vi "Sweep - Create Tasks.vi"(8 "error in (no error)":errorcluster, 11 "measurement configuration":T3={"digital channel list"="", "frame clock rate"=0.0, "number of channels"=0, "channel length"=0, "bit depth"=0, "data justification"=enum."Left Justified", "endianness"=enum."MSB First", "bit clock edge sync"=enum."Rising", "frame sync edge for channel 0"=enum."Rising", "channel 0 offset"=0, "master clock channel list"="", "master clock rate"=0.0, "enable dither"=FALSE, "logic level"=enum."3.3 V", "signal frequency"=1000.0, "output level"=0.0, "output level units"=enum."% FS", "output range (pk-pk)"=0.0, "load impedance"=0.0, "signal phase"=0.0, "acq sampling rate"=0.0, "min measurement cycles"=0, "min measurement time (s)"=0.0, "min settling cycles"=0, "min settling time (s)"=0.0, "acq channel"="", "band start"=0.0, "band stop"=0.0, "weighting filter"=enum."Linear", "highpass filter"=enum."DC", "lowpass filter"=enum."No filter", "SNR units"=enum."dB", "THD+N units"=enum."dB", "THD units"=enum."dB", "gain units"=enum."dB"} {"signal phase" format="%0.2f"; "master clock rate" format="%#_6pHz"; "frame clock rate" format="%#_6pHz"}) -> (0 "error out":errorcluster, 2 "DAQmx task":refnum<k21>, 3 "PCM tasks":T1)   [LabVIEW 2023]
uses:
  controls/single tone measurement settings (HW).ctl
  controls/digital audio protocol/data justification.ctl
  controls/digital audio protocol/endianness.ctl
  controls/digital audio protocol/digital edge.ctl
  controls/digital audio protocol/logic level.ctl
  controls/digital output level units.ctl
  controls/weighting filter.ctl
  controls/highpass filter.ctl
  controls/lowpass filter.ctl
  controls/units - snr.ctl
  controls/units - ratio.ctl
  controls/digital audio protocol/PCM tasks.ctl
  <vilib>/PDM Acquisition Toolkit/host/Classes/Tasks/PCM Output/Controls/PCM Output Task DVR.ctl
  <vilib>/PDM Acquisition Toolkit/host/Classes/Tasks/PCM Output/PCM Output Task.lvclass
  <vilib>/PDM Acquisition Toolkit/shared/controls/clock mode.ctl
  <vilib>/PDM Acquisition Toolkit/shared/controls/PCM Frame Sync Control.ctl
  <vilib>/PDM Acquisition Toolkit/shared/controls/Digital Edge.ctl
  <vilib>/PDM Acquisition Toolkit/shared/controls/PCM Data Format Configuration.ctl
  <vilib>/PDM Acquisition Toolkit/shared/controls/PCM Bit Endianness.ctl
  <vilib>/PDM Acquisition Toolkit/shared/controls/PCM Data Justification.ctl
  <vilib>/DAQmx/create/channels.llb/DAQmx Create Channel (AI-Voltage-Basic).vi
  <vilib>/DAQmx/configure/timing.llb/DAQmx Timing (Sample Clock).vi
  <vilib>/PDM Acquisition Toolkit/host/API/Public/Function Generator/Configure Custom Signal (N Ch) - PCM Output Task.vi
  <vilib>/PDM Acquisition Toolkit/shared/PDM Shared.lvlib
  <vilib>/PDM Acquisition Toolkit/host/API/PDM Acquisition Toolkit.lvlib
  controls/audio controls.lvlib
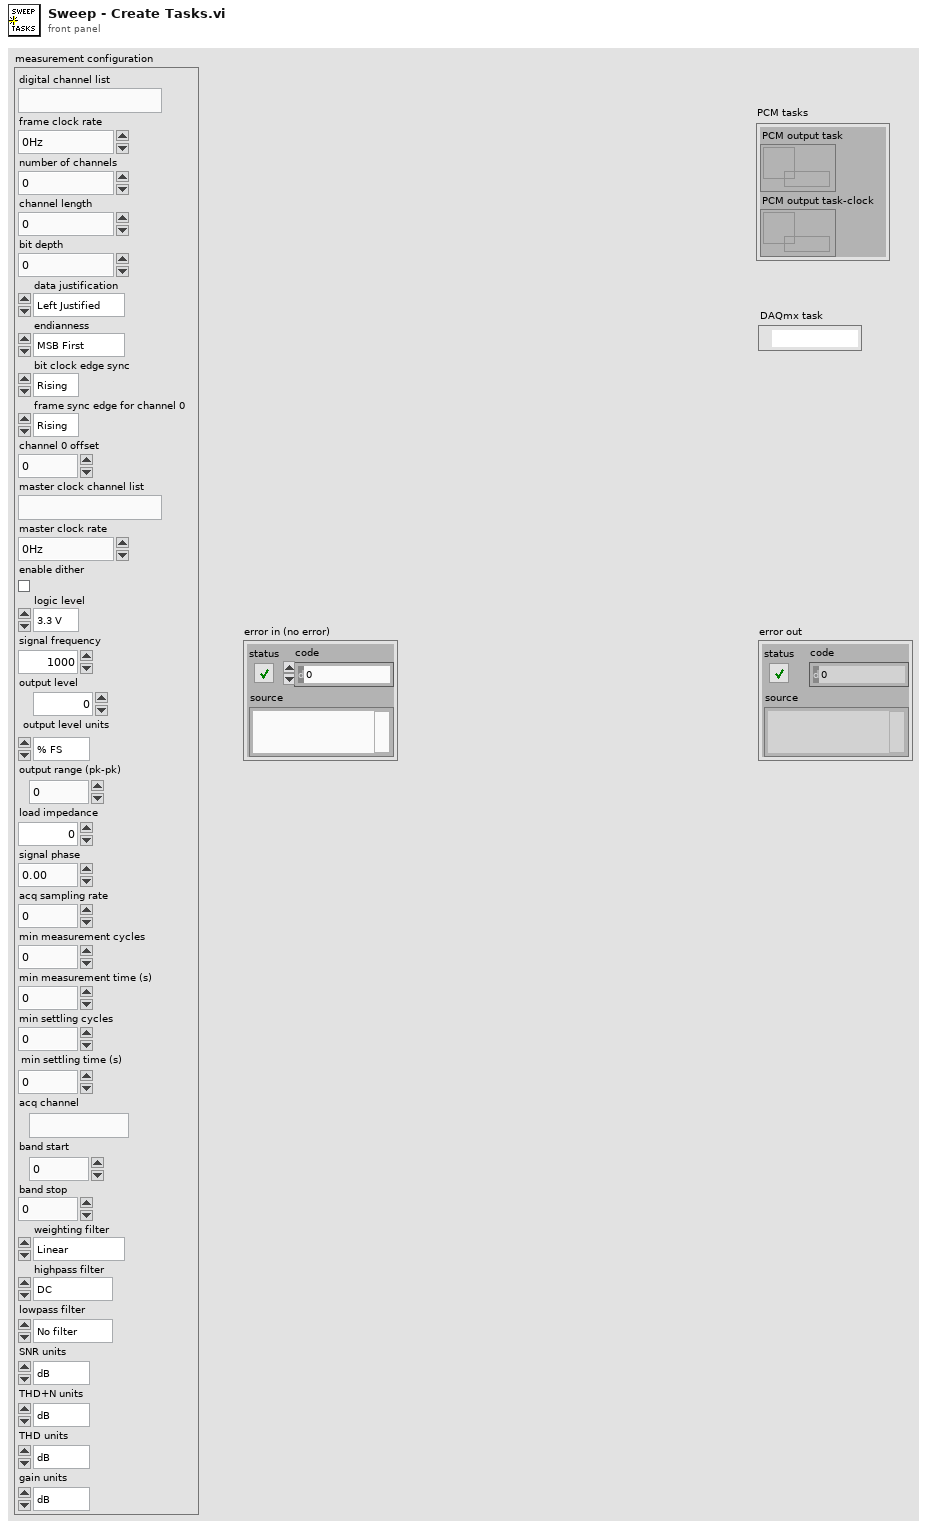
[diagram p1: front panel]
types:
  T1 = typedef "PCM tasks.ctl" = cluster{"PCM output task":T2, "PCM output task-clock":T2}
  T2 = typedef "PDM Acquisition Class Library.lvlib/PCM Output Task.lvclass/PCM Output Task DVR.ctl" = refnum<data-value>
  T3 = typedef "single tone measurement settings (HW).ctl" = cluster{"digital channel list":string, "frame clock rate":dbl, "number of channels":u32, "channel length":u32, "bit depth":u32, "data justification":T4, "endianness":T5, "bit clock edge sync":T6, "frame sync edge for channel 0":T6, "channel 0 offset":u32, "master clock channel list":string, "master clock rate":dbl, "enable dither":bool, "logic level":T7, "signal frequency":dbl, "output level":dbl, "output level units":T8, "output range (pk-pk)":dbl, "load impedance":dbl, "signal phase":dbl, "acq sampling rate":dbl, "min measurement cycles":u32, "min measurement time (s)":dbl, "min settling cycles":u32, "min settling time (s)":dbl, "acq channel":string, "band start":dbl, "band stop":dbl, "weighting filter":T9, "highpass filter":T10, "lowpass filter":T11, "SNR units":T12, "THD+N units":T13, "THD units":T13, "gain units":T13}
  T4 = typedef "data justification.ctl" = enum32{"Left Justified", "Right Justified"}
  T5 = typedef "endianness.ctl" = enum32{"MSB First", "LSB First"}
  T6 = typedef "digital edge.ctl" = enum32{"Rising", "Falling"}
  T7 = typedef "logic level.ctl" = enum32{"3.3 V", "1.8 V", "1.2 V"}
  T8 = typedef "audio controls.lvlib/digital output level units.ctl" = enum32{"% FS", "dBFS", "V"}
  T9 = typedef "weighting filter.ctl" = enum32{"Linear", "A-weighting", "B-weighting", "C-weighting"}
  T10 = typedef "highpass filter.ctl" = enum32{"DC", "AC"}
  T11 = typedef "lowpass filter.ctl" = enum32{"No filter", "AES17 20kHz", "AES17 40kHz"}
  T12 = typedef "audio controls.lvlib/units - snr.ctl" = enum32{"dB", "x/y"}
  T13 = typedef "audio controls.lvlib/units - ratio.ctl" = enum32{"dB", "%", "x/y"}
  T14 = typedef "PDM Shared.lvlib/PCM Data Format Configuration.ctl" = cluster{"Frame Sync Edge for Channel 0":T15, "Channel Count Per Frame":u8, "Channel Length":u16, "Bit Depth":u8, "Channel 0 Offset":u16, "Endianness":T16, "Data Justification":T17}
  T15 = typedef "PDM Shared.lvlib/Digital Edge.ctl" = enum8{"Rising", "Falling"}
  T16 = typedef "PDM Shared.lvlib/PCM Bit Endianness.ctl" = enum16{"MSB First", "LSB First"}
  T17 = typedef "PDM Shared.lvlib/PCM Data Justification.ctl" = enum16{"Left Justified", "Right Justified"}
  T18 = typedef "PDM Shared.lvlib/PCM Frame Sync Control.ctl" = cluster{"Frame Length":u16, "Frame Sync Pulse Width":u16, "Bit Clock Edge  Sync":T15}
  T19 = typedef "PDM Shared.lvlib/clock mode.ctl" = enum16{"divided clock", "DDS"}
  T20 = typedef "PDM Acquisition Class Library.lvlib/I2S Output Task.lvclass/SignalProperties.ctl" = cluster{"cyclic signal":dbl[], "channel parameters":T21[]}
  T21 = typedef "PDM Acquisition Class Library.lvlib/I2S Output Channel.lvclass/GenerationChannelProperties.ctl" = cluster{"cyclic period":dbl, "cyclic phase offset":dbl, "gain":dbl}
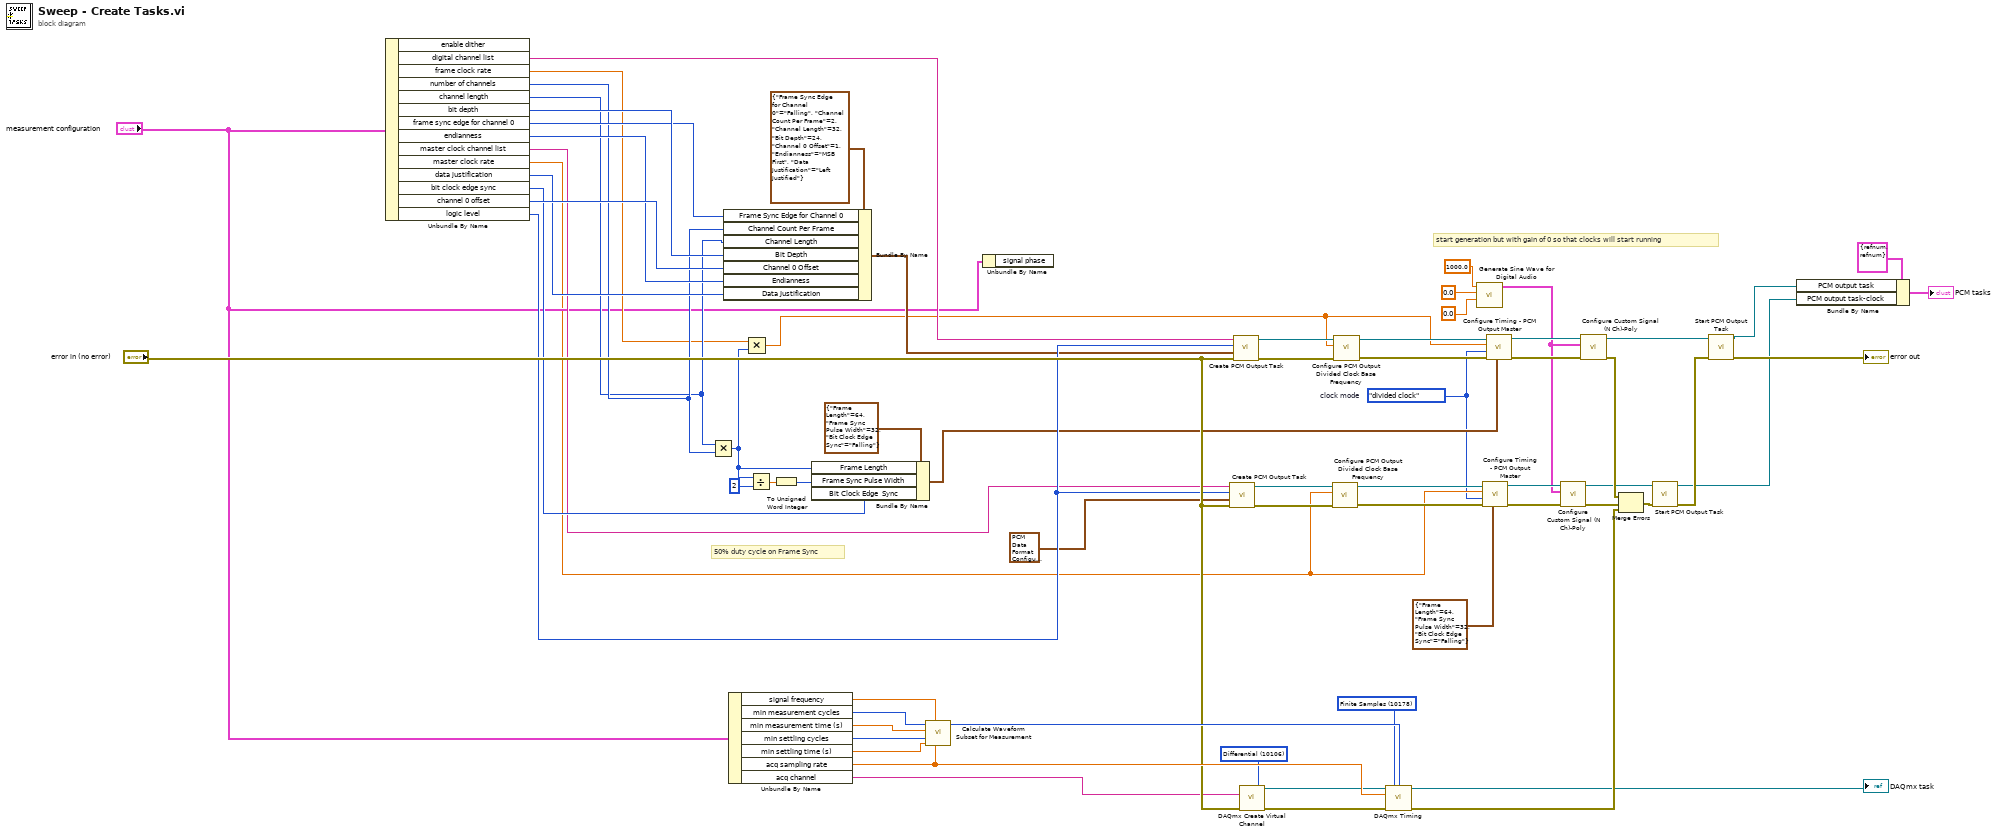
[diagram p0: block diagram]
diagram:
  w51 = 10106 items=["Default"=-1, "RSE"=10083, "NRSE"=10078, "Differential"=10106, "Pseudodifferential"=12529] ("input terminal configuration")
  w45 = 10178 items=["Finite Samples"=10178, "Continuous Samples"=10123, "Hardware Timed Single Point"=12522] ("sample mode")
  w1 = clock_mode."divided clock"  # clock mode
  # "start generation but with gain of 0 so that clocks will start running"
  # "50% duty cycle on Frame Sync"
  n1 = Unbundle By Name("measurement configuration") -> ("digital channel list"=w58:string, "frame clock rate"=w46:dbl, "number of channels"=w48:u32, "channel length"=w47:u32, "bit depth"=w68:u32, "frame sync edge for channel 0"=w53:T6, "endianness"=w54:T5, "master clock channel list"=w49:string, "master clock rate"=w2:dbl, "data justification"=w52:T4, "bit clock edge sync"=w55:T6, "channel 0 offset"=w56:u32, "logic level"=w57:T7)  [unwired: 1 out]
  n2 = Multiply(x=w47, y=w48) -> (x*y=w33:u32)
  n3 = Bundle By Name(cluster=T14 {"Frame Sync Edge for Channel 0"=enum."Falling", "Channel Count Per Frame"=2, "Channel Length"=32, "Bit Depth"=24, "Channel 0 Offset"=1, "Endianness"=enum."MSB First", "Data Justification"=enum."Left Justified"} ("PCM Data Configuration"), "Frame Sync Edge for Channel 0"=w53, "Channel Count Per Frame"=w48, "Channel Length"=w47, "Bit Depth"=w68, "Channel 0 Offset"=w56, "Endianness"=w54, "Data Justification"=w52) -> (w35:T14)
  n4 = Unbundle By Name("measurement configuration") -> ("signal frequency"=w12:dbl, "min measurement cycles"=w64:u32, "min measurement time (s)"=w65:dbl, "min settling cycles"=w66:u32, "min settling time (s)"=w67:dbl, "acq sampling rate"=w62:dbl, "acq channel"=w50:string)
  n5 = Multiply(x=w46, y=w33) -> (x*y=w7:dbl)
  n6 = Divide(x=w33, y=u16 2) -> (x/y=w31:dbl)
  n7 = To Unsigned Word Integer(number=w31) -> (unsigned 16bit integer=w32:u16)
  n8 = Bundle By Name(cluster=T18 {"Frame Length"=64, "Frame Sync Pulse Width"=32, "Bit Clock Edge  Sync"=enum."Falling"} ("Frame Sync Clock Control"), "Frame Length"=w33, "Frame Sync Pulse Width"=w32, "Bit Clock Edge  Sync"=w55) -> (w29:T18)
  n9 = call "Calculate Waveform Subset for Measurement.vi"("sampling rate"=w62, "signal frequency"=w12, "minimum settling duration"=w67, "minimum settling cycles"=w66, "minimum measurement duration"=w65, "minimum measurement cycles"=w64) -> ("total acquisition (samples)"=w63:u32)  [unwired: 3 in, 2 out]
  n10 = Unbundle By Name("measurement configuration") -> ()  [unwired: 1 out]
  n11 = call <vilib>:"Create PCM Output Task.vi"("error in"="error in (no error)", "PCM data configuration"=T14 {"Frame Sync Edge for Channel 0"=enum."Falling", "Channel Count Per Frame"=2, "Channel Length"=32, "Bit Depth"=24, "Channel 0 Offset"=1, "Endianness"=enum."MSB First", "Data Justification"=enum."Left Justified"} ("PCM Data Configuration 2"), "logic level"=w57, "channel list"=w49) -> ("error out"=w5:errorcluster, "PCM output task out"=w6:T2)  [unwired: 6 in]
  n12 = call <vilib>:"Create PCM Output Task.vi"("error in"="error in (no error)", "PCM data configuration"=w35, "logic level"=w57, "channel list"=w58) -> ("error out"=w10:errorcluster, "PCM output task out"=w11:T2)  [unwired: 6 in]
  n13 = call-poly <vilib>:"DAQmx Create Virtual Channel.vi"("input terminal configuration"=w51, "physical channels"=w50, "error in"="error in (no error)") -> ("task out"=w43:refnum<k21>, "error out"=w42:errorcluster)  [unwired: 11 in]
  n14 = call <vilib>:"Configure PCM Output Divided Clock Base Frequency.vi"("error in"=w5, "Bit Clock rate"=w2, "PCM output task in"=w6) -> ("error out"=w3:errorcluster, "PCM output task out"=w4:T2)  [unwired: 7 in]
  n15 = call <vilib>:"Configure PCM Output Divided Clock Base Frequency.vi"("error in"=w10, "Bit Clock rate"=w7, "PCM output task in"=w11) -> ("error out"=w8:errorcluster, "PCM output task out"=w9:T2)  [unwired: 7 in]
  n16 = call-poly <vilib>:"DAQmx Timing.vi"("task/channels in"=w43, "sample mode"=w45, "samples per channel"=w63, "rate"=w62, "error in"=w42) -> ("task out"=→"DAQmx task":refnum<k21>, "error out"=w44:errorcluster)  [unwired: 9 in]
  n17 = call "Generate Sine Wave for Digital Audio.vi"("phase"=0.0, "gain"=0.0, "frequency"=1000.0) -> ("Signal Properties"=w20:T20)  [unwired: 8 in]
  n18 = call <vilib>:"Configure Timing - PCM Output Master.vi"("Frame Sync Clock Control"=T18 {"Frame Length"=64, "Frame Sync Pulse Width"=32, "Bit Clock Edge  Sync"=enum."Falling"} ("Frame Sync Clock Control 2"), "error in"=w3, "clock mode"=w1, "Bit Clock rate"=w2, "PCM output task in"=w4) -> ("error out"=w36:errorcluster, "PCM output task out"=w37:T2)  [unwired: 4 in, 1 out]
  n19 = call <vilib>:"Configure Timing - PCM Output Master.vi"("Frame Sync Clock Control"=w29, "error in"=w8, "clock mode"=w1, "Bit Clock rate"=w7, "PCM output task in"=w9) -> ("error out"=w60:errorcluster, "PCM output task out"=w59:T2)  [unwired: 4 in, 1 out]
  n20 = call-poly <vilib>:"Configure Custom Signal (N Ch)-Poly.vi"("error in"=w36, "signal parameters"=w20, "PCM output task in"=w37) -> ("error out"=w41:errorcluster, "PCM output task out"=w38:T2)  [unwired: 7 in]
  n21 = call-poly <vilib>:"Configure Custom Signal (N Ch)-Poly.vi"("error in"=w60, "signal parameters"=w20, "PCM output task in"=w59) -> ("error out"=w40:errorcluster, "PCM output task out"=w39:T2)  [unwired: 7 in]
  n22 = Merge Errors(w40, w41, w44) -> (w27:errorcluster)
  n23 = call <vilib>:"Start PCM Output Task.vi"("error in"=w27, "PCM output task in"=w38) -> ("error out"=w26:errorcluster, "PCM output task out"=w13:T2)  [unwired: 8 in]
  n24 = call <vilib>:"Start PCM Output Task.vi"("error in"=w26, "PCM output task in"=w39) -> ("error out"=→"error out":errorcluster, "PCM output task out"=w14:T2)  [unwired: 8 in]
  n25 = Bundle By Name(cluster=T1 {"PCM output task"=refnum, "PCM output task-clock"=refnum} ("PCM tasks"), "PCM output task"=w14, "PCM output task-clock"=w13) -> (→"PCM tasks":T1)
